vi "Pockels Cal-Check conditions match.vi"() -> (2 "Continue":bool)   [LabVIEW 2013]
uses:
  Typedefs/Which path.ctl
  Globals/gl_Calibration globals.vi
  Program Files (x86)/National Instruments/LabVIEW 2013/user.lib/My Palettes.lib/Files & paths/Spreadsheet/Read From Spreadsheet File (string)-Mod.vi
panel:
  out "Wavelength value":dbl
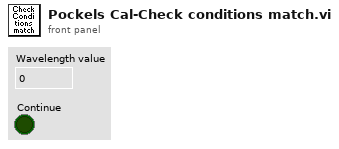
[diagram p1: front panel]
types:
  T1 = typedef "Which path.ctl" = enum16{"Configuration Files", "Calibration Files", "Images", "Setup.ini", "Loaded User profile.ini", "User's-Previous session.ini", "New user profile.ini", "Selected User profile.ini", "User profiles folder", "Power meter scaling.txt", "FOV Cal.ini"}
  T2 = enum16{"Continue anyway", "Conditions match", "Conditions mismatch"}
  T3 = typedef "Pockels cal conditions cluster.ctl" = cluster{"Wavelength":u16, "Zoom":u8, "Dwell time (us)":dbl, "Pockels bias":i16, "Prism 1":u16, "Prism 2":u16, "Laser power during pockels cal (mW)":u16}
  T4 = cluster{"Pockels cal.Zoom":u8, "Pockels cal.Dwell time (µs)":dbl}
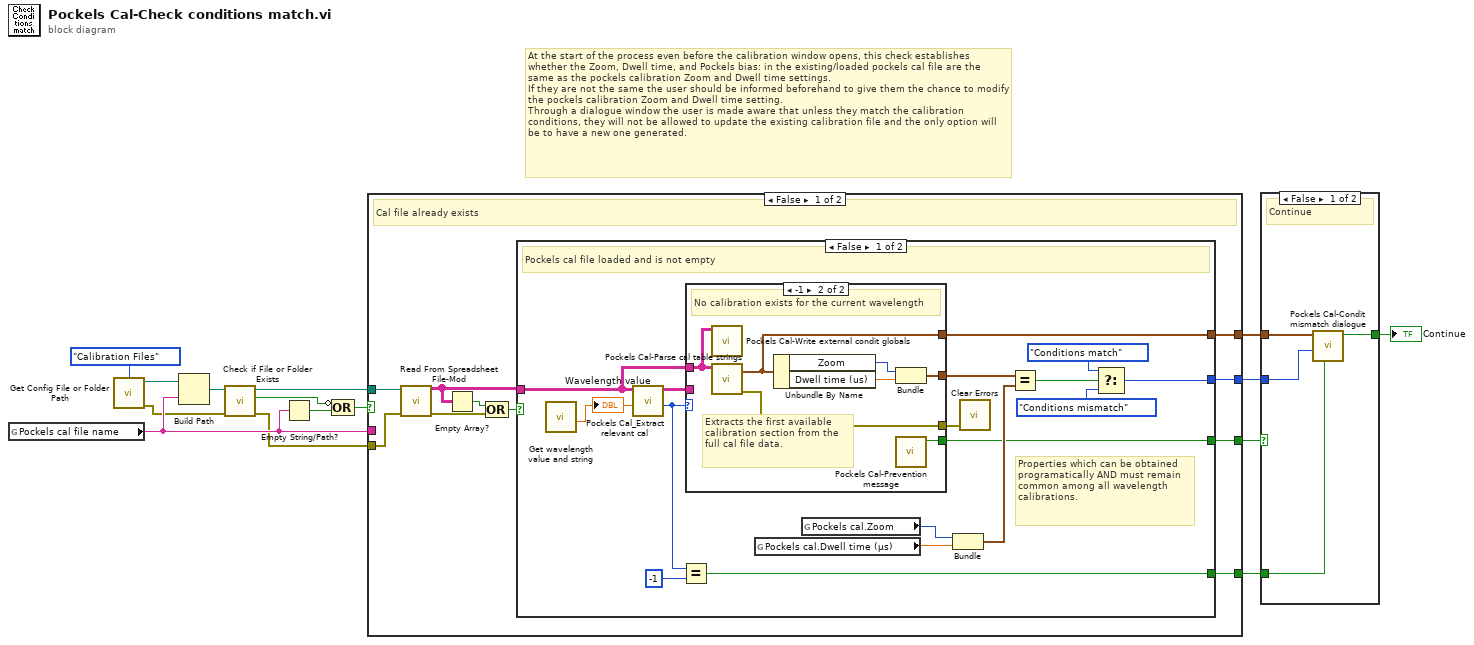
[diagram p0: block diagram]
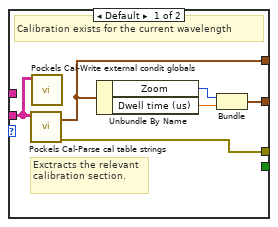
[diagram p3: hidden frame]
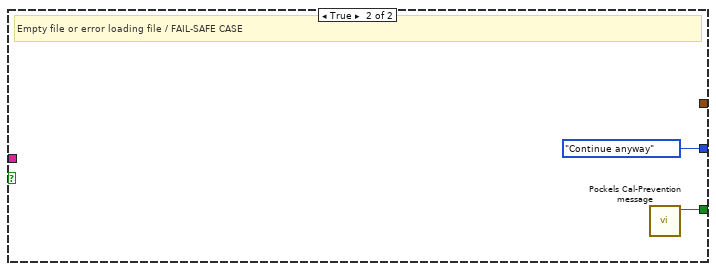
[diagram p4: hidden frame]
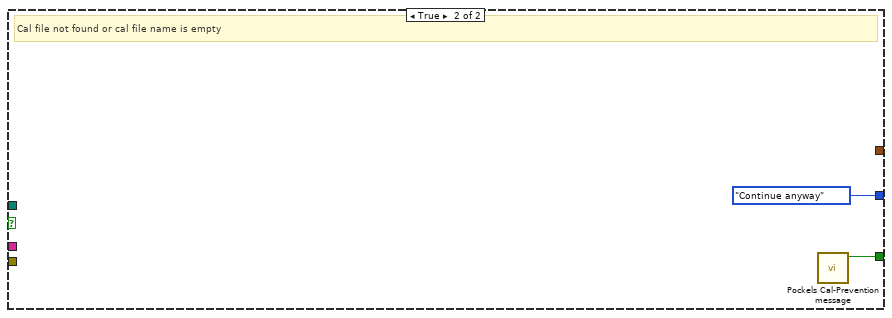
[diagram p5: hidden frame]
diagram:
  # "At the start of the process even before the calibration window opens, this check establishes whether the Zoom, Dwell time, and Pockels bias: in the existing/loaded pockels cal file are the same as the pockels calibration Zoom and Dwell time settings. \nIf they are not the same the user should be informed beforehand to give them the chance to modify the pockels calibration Zoom and Dwell time setting.\nThrough a dialogue window the user is made aware that unless they match the calibration conditions, they will not be allowed to update the existing calibration file and the only option will be to have a new one generated."
  n1 = global read "gl_Calibration globals.vi" "Pockels cal file name"() -> (w12:string)
  n2 = call "Get Config File or Folder Path.vi"("Which file or folder?"=Which_path."Calibration Files" ("Which path?")) -> ("Error Out"=w6:errorcluster, "File Path"=w15:path)  [unwired: 8 in, 1 out]
  n3 = Build Path(base path=w15, name or relative path=w12) -> (appended path=w13:path)
  n4 = call <vilib>:"Check if File or Folder Exists.vi"("error in (no error)"=w6, "path"=w13) -> ("error out"=w7:errorcluster, "file or folder exists?"=w11:bool, "dup path"=w8:path)  [unwired: 7 in]
  n5 = Empty String/Path?(string/path=w12) -> (empty?=w10:bool)
  n6 = Compound Arithmetic op=OR(invert w11, w10) -> (w9:bool)
  n7 = case shown="False" w9 {
    tunnel: w8 -> [w23 _]
    tunnel: w12 -> [_ _]
    tunnel: [w22 T2."Continue anyway" ("Function")] -> w4
    tunnel: w7 -> [w21 _]
    tunnel: [w20 _] -> w3
    tunnel: [w17 _] -> w2
    tunnel: [w16 w58] -> w1
    frame False {
      # "Cal file already exists"
      n8 = call-poly "Read From Spreadsheet File-Mod.vi"("file path (dialog if empty)"=w23, "error in"=w21) -> ("all rows"=w18:string[][], "error out"=w19:errorcluster)  [unwired: 8 in, 4 out]
      n9 = Empty Array?(array=w18) -> (empty?=w24:bool)
      n10 = Compound Arithmetic op=OR(w24, w19) -> (w25:bool)
      n11 = case shown="False" w25 {
        tunnel: w18 -> [w40 _]
        tunnel: [w32 T2."Continue anyway" ("Function")] -> w22
        tunnel: [w42 _] -> w20
        tunnel: [w27 _] -> w17
        tunnel: [w26 w56] -> w16
        frame False {
          # "Properties which can be obtained programatically AND must remain common among all wavelength calibrations."
          # "Pockels cal file loaded and is not empty"
          n12 = call "Get wavelength value and string.vi"() -> ("Wavelength value"=w31:dbl)  [unwired: 9 in, 2 out]
          "Wavelength value" <- w31
          n13 = call "Pockels Cal_Extract relevant cal.vi"("Wavelength value"=w31, "Loaded table"=w40) -> ("Index of replacement"=w29:i32, "Relevant cal only"=w41:string[][])  [unwired: 6 in, 2 out]
          n14 = Equal?(x=w29, y=-1) -> (x = y?=w27:bool)
          n15 = case shown="-1" w29 {
            tunnel: [w48 w55] -> w42
            tunnel: w41 -> [w43 _]
            tunnel: w40 -> [_ w50]
            tunnel: [w45 w52] -> w35
            tunnel: [w44 w51] -> w30
            tunnel: [_ w49] -> w26
            frame Default {
              # "Exctracts the relevant calibration section."
              # "Calibration exists for the current wavelength"
              n16 = call "Pockels Cal-Parse cal table strings.vi"("SINGLE CAL SET (inc. headers & info)"=w43) -> ("error out"=w44:errorcluster, "Cal conditions"=w48:T3)  [unwired: 5 in, 4 out]
              n17 = call "Pockels Cal-Write external condit globals.vi"("Pockels Cal table"=w43) -> ()  [unwired: 11 in]
              n18 = Unbundle By Name(w48) -> ("Zoom"=w47:u8, "Dwell time (us)"=w46:dbl)
              n19 = Bundle("Zoom"=w47, "Dwell time (us)"=w46) -> (w45:cluster{"Zoom":u8, "Dwell time (us)":dbl})  [unwired: 1 in]
            }
            frame -1 {
              # "Extracts the first available calibration section from the full cal file data."
              # "No calibration exists for the current wavelength"
              n20 = call "Pockels Cal-Write external condit globals.vi"("Pockels Cal table"=w50) -> ()  [unwired: 11 in]
              n21 = call "Pockels Cal-Parse cal table strings.vi"("SINGLE CAL SET (inc. headers & info)"=w50) -> ("error out"=w51:errorcluster, "Cal conditions"=w55:T3)  [unwired: 5 in, 4 out]
              n22 = Unbundle By Name(w55) -> ("Zoom"=w54:u8, "Dwell time (us)"=w53:dbl)
              n23 = Bundle("Zoom"=w54, "Dwell time (us)"=w53) -> (w52:cluster{"Zoom":u8, "Dwell time (us)":dbl})  [unwired: 1 in]
              n24 = call "Pockels Cal-Prevention message.vi"() -> ("Cancel"=w49:bool)  [unwired: 11 in]
            }
          }
          n25 = global read "gl_Calibration globals.vi" "Pockels cal.Dwell time (µs)"() -> (w38:dbl)
          n26 = global read "gl_Calibration globals.vi" "Pockels cal.Zoom"() -> (w39:u8)
          n27 = Bundle("Pockels cal.Zoom"=w39, "Pockels cal.Dwell time (µs)"=w38) -> (w37:T4)  [unwired: 1 in]
          n28 = call <vilib>:"Clear Errors.vi"("error in (no error)"=w30) -> ()  [unwired: 6 in, 1 out]
          n29 = Equal?(x=w35, y=w37) -> (x = y?=w36:bool)
          n30 = Select(t=T2."Conditions match" ("Function"), s=w36, f=T2."Conditions mismatch" ("Function")) -> (s? t:f=w32:T2)
        }
        frame True {
          # "Empty file or error loading file / FAIL-SAFE CASE"
          n31 = call "Pockels Cal-Prevention message.vi"() -> ("Cancel"=w56:bool)  [unwired: 11 in]
        }
      }
    }
    frame True {
      # "Cal file not found or cal file name is empty"
      n32 = call "Pockels Cal-Prevention message.vi"() -> ("Cancel"=w58:bool)  [unwired: 11 in]
    }
  }
  n33 = case shown="False" w1 {
    tunnel: [w63 _] -> w5
    tunnel: w4 -> [w62 _]
    tunnel: w3 -> [w61 _]
    tunnel: w2 -> [w60 _]
    frame False {
      # "Continue"
      n34 = call "Pockels Cal-Condit mismatch dialogue.vi"("New cal section to be added"=w60, "Function"=w62, "Cal conditions"=w61) -> ("Continue?"=w63:bool)  [unwired: 7 in, 1 out]
    }
    frame True {
      # "Aborted"
    }
  }
  "Continue" <- w5
